vi "Modbus register.vi"(4 "State":i16=-1, 5 "Time":dbl format="%.2f", 6 "Sensor Values":dbl[](array[numeric]), 7 "Set Points":dbl[](array[numeric])=[0.0]) -> (0 "required data":T2={"Set Point names"=["Device ID", "register"], "required number of setpoints"=2, "required number of sensors"=0, "Sensor names"=[]}, 3 "output value":dbl)   [LabVIEW 2019]
uses:
  modbusrtu/MB ID-Address.ctl
  modbusrtu/MB cmd buffer.ctl
panel:
  in  "MB ID-Address in":T1
  # "Enter the correct information for this control code in the required data structure below. Then make the current value default by right clicking on the border of the data structure. Select \"data operations\" and then select \"make current value default\". These values will be displayed by process controller."
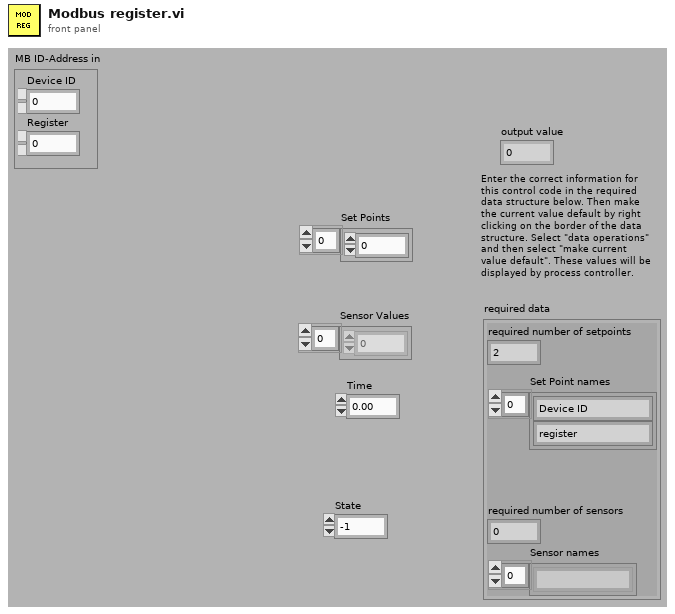
[diagram p1: front panel]
types:
  T1 = typedef "MB ID-Address.ctl" = cluster{"Device ID":u8, "Register":u16}
  T2 = cluster{"Set Point names":string[], "required number of setpoints":u8, "required number of sensors":u8, "Sensor names":string[]}
  T3 = cluster{"Set Points[0]":dbl, "Set Points[1]":dbl}
  T4 = typedef "MB cmd buffer.ctl" = enum16{"ProCoDA", "MB succeed", "MB error", "MB Next Task", "ProCoDA read 1", "Commands pending"}
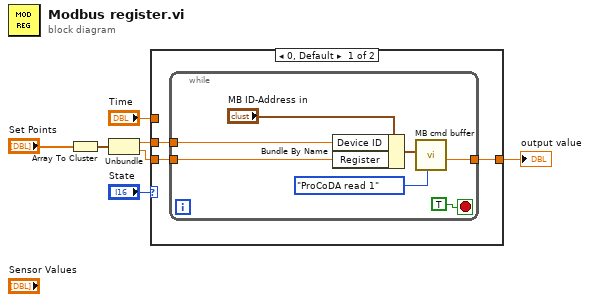
[diagram p0: block diagram]
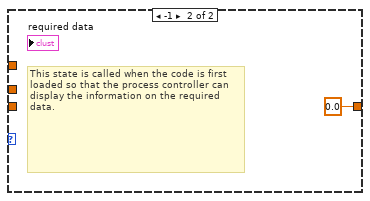
[diagram p2: hidden frame]
diagram:
  n1 = Array To Cluster(array="Set Points") -> (cluster=w3:T3)
  n2 = Unbundle(w3) -> ("Set Points[0]"=w2:dbl, "Set Points[1]"=w1:dbl)
  n3 = case shown="0, Default" "State" {
    tunnel: [w10 0.0 ("fraction on")] -> w6
    tunnel: "Time" -> [_ _]
    tunnel: w2 -> [w9 _]
    tunnel: w1 -> [w8 _]
    frame 0, Default {
      n4 = while {
        tunnel: [w16] -> w10
        tunnel: w9 -> [w13]
        tunnel: w8 -> [w11]
        stop <- TRUE stop-if-true
        n5 = Bundle By Name(cluster="MB ID-Address in", "Device ID"=w13, "Register"=w11) -> (w14:T1)
        n6 = call "MB cmd buffer.vi"("MB cmd buffer"=MB_cmd_buffer."ProCoDA read 1", "MB ID-Address in"=w14) -> ("output value"=w16:dbl)  [unwired: 3 in, 6 out]
      }
    }
    frame -1 {
      # "This state is called when the code is first loaded so that the process controller can display the information on the required data."
    }
  }
  "output value" <- w6
